vi "Keithley 2100 Series Fetch Multiple.vi"() -> ()   [LabVIEW 2020]
doc: "This example shows how to select a function and fetch multiple measurements."
uses:
  Public/Configure/Configure DC Volts.vi
  Public/Configure/Configure AC Volts.vi
  Public/Configure/Configure DC Current.vi
  Public/Configure/Configure AC Current.vi
  Public/Configure/Configure 2 Wire Resistance.vi
  Public/Configure/Configure 4 Wire Resistance.vi
  Keithley 2100 Series.lvlib
panel:
  out "Measurements":dbl[](array[numeric])
  in  "Timeout (10000 ms)":i32=10000 format="%#.6g"
  in  "Sample Count (1)":i32=1 min=1 max=50000
  in  "Function (0: DC Volts)":u16(ring) items=["DC Volts", "AC Volts", "DC Current", "AC Current", "2-Wire Resistance", "4-Wire Resistance"]
  in  "VISA resource name":refnum<visa-resource-name>="GPIB::16"
  # "This example shows how to select a function, \nuse a bus trigger, and read multiple measurements.\n\nInstructions:\n1. Select a VISA resource name,function,Sample Count\n and appropriate timeout.\n2. Run the VI."
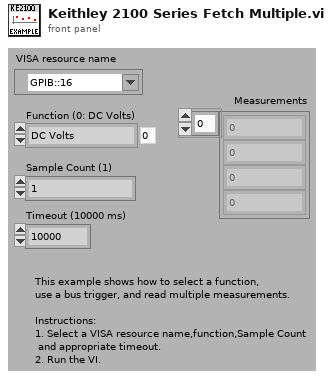
[diagram p1: front panel]
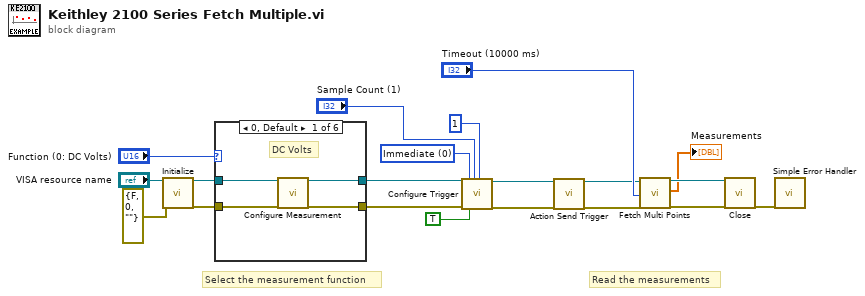
[diagram p0: block diagram]
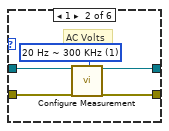
[diagram p2: hidden frame]
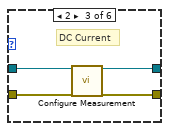
[diagram p3: hidden frame]
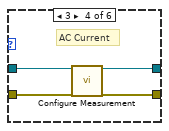
[diagram p4: hidden frame]
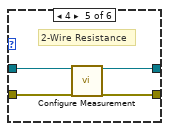
[diagram p5: hidden frame]
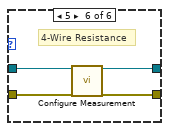
[diagram p6: hidden frame]
diagram:
  w2 = u16 0 items=["Immediate", "Bus", "External"] ("Source (0: Immediate)")
  # "Read the measurements"
  # "Select the measurement function"
  n1 = call "Initialize.vi"("VISA resource name"="VISA resource name", "error in (no error)"=errorcluster {"status"=FALSE, "code"=0, "source"=""}) -> ("VISA resource name out"=w19:refnum<visa-resource-name>, "error out"=w20:errorcluster)  [unwired: 16 in]
  n2 = case shown="0, Default" "Function (0: DC Volts)" {
    tunnel: w20 -> [w24 w29 w33 w37 w41 w45]
    tunnel: w19 -> [w23 w28 w32 w36 w40 w44]
    tunnel: [w22 w27 w31 w35 w39 w43] -> w5
    tunnel: [w21 w26 w30 w34 w38 w42] -> w6
    frame 0, Default {
      # "DC Volts"
      n3 = call-poly "Configure Measurement.vi"("VISA resource name"=w23, "error in (no error)"=w24) -> ("VISA resource name out"=w21:refnum<visa-resource-name>, "error out"=w22:errorcluster)  [unwired: 16 in]
    }
    frame 1 {
      w25 = u16 1 items=["3 Hz ~ 300 KHz", "20 Hz ~ 300 KHz", "200 Hz ~ 300 KHz"] ("Bandwidth (20 Hz)")
      # "AC Volts"
      n4 = call-poly "Configure Measurement.vi"("VISA resource name"=w28, "error in (no error)"=w29, "Bandwidth (20 Hz)"=w25) -> ("VISA resource name out"=w26:refnum<visa-resource-name>, "error out"=w27:errorcluster)  [unwired: 15 in]
    }
    frame 2 {
      # "DC Current"
      n5 = call-poly "Configure Measurement.vi"("VISA resource name"=w32, "error in (no error)"=w33) -> ("VISA resource name out"=w30:refnum<visa-resource-name>, "error out"=w31:errorcluster)  [unwired: 16 in]
    }
    frame 3 {
      # "AC Current"
      n6 = call-poly "Configure Measurement.vi"("VISA resource name"=w36, "error in (no error)"=w37) -> ("VISA resource name out"=w34:refnum<visa-resource-name>, "error out"=w35:errorcluster)  [unwired: 16 in]
    }
    frame 4 {
      # "2-Wire Resistance"
      n7 = call-poly "Configure Measurement.vi"("VISA resource name"=w40, "error in (no error)"=w41) -> ("VISA resource name out"=w38:refnum<visa-resource-name>, "error out"=w39:errorcluster)  [unwired: 16 in]
    }
    frame 5 {
      # "4-Wire Resistance"
      n8 = call-poly "Configure Measurement.vi"("VISA resource name"=w44, "error in (no error)"=w45) -> ("VISA resource name out"=w42:refnum<visa-resource-name>, "error out"=w43:errorcluster)  [unwired: 16 in]
    }
  }
  n9 = call "Configure Trigger.vi"("VISA resource name"=w6, "error in (no error)"=w5, "Source (0: Immediate)"=w2, "Auto Delay? (T: Auto)"=TRUE, "Sample Count (1)"="Sample Count (1)", "Trigger Count (1)"=1) -> ("VISA resource name out"=w8:refnum<visa-resource-name>, "error out"=w7:errorcluster)  [unwired: 12 in]
  n10 = call "Action Send Trigger.vi"("VISA resource name"=w8, "error in (no error)"=w7) -> ("VISA resource name out"=w10:refnum<visa-resource-name>, "error out"=w9:errorcluster)  [unwired: 16 in]
  n11 = call "Fetch Multi Points.vi"("VISA resource name"=w10, "Timeout (10000 ms)"="Timeout (10000 ms)", "error in (no error)"=w9) -> ("VISA resource name out"=w13:refnum<visa-resource-name>, "Measurements"=→"Measurements":dbl[], "error out"=w14:errorcluster)  [unwired: 14 in]
  n12 = call "Close.vi"("VISA resource name"=w13, "error in (no error)"=w14) -> ("error out"=w18:errorcluster)  [unwired: 17 in]
  n13 = call <vilib>:"Simple Error Handler.vi"("error in (no error)"=w18) -> ()  [unwired: 4 in, 5 out]
